vi "CalculateAverageDPARate.vi"(8 "Duration (sec)":dbl, 9 "Period (sec)":dbl, 10 "DPA Rate":dbl, 11 "Total DPA Rate In":dbl) -> (2 "Average DPA Rate":dbl, 3 "Total DPA Rate Out":dbl)   [LabVIEW 2012]
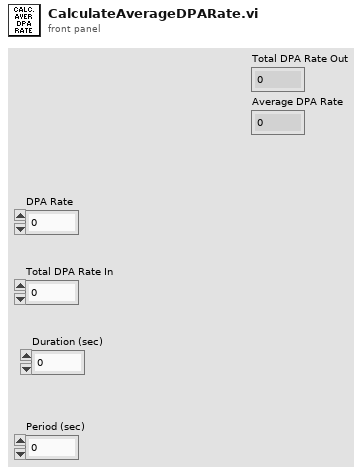
[diagram p1: front panel]
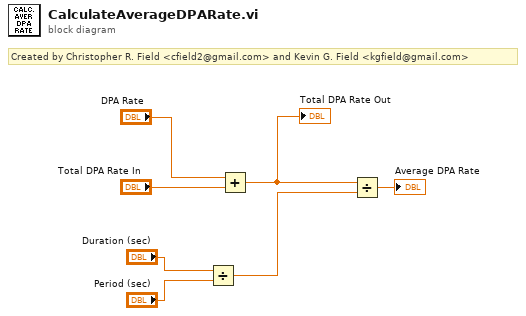
[diagram p0: block diagram]
diagram:
  # "Created by Christopher R. Field <cfield2@gmail.com> and Kevin G. Field <kgfield@gmail.com>"
  n1 = Divide(x="Duration (sec)", y="Period (sec)") -> (x/y=w2:dbl)
  n2 = Add(x="DPA Rate", y="Total DPA Rate In") -> (x+y=w3:dbl)
  "Total DPA Rate Out" <- w3
  n3 = Divide(x=w3, y=w2) -> (x/y=→"Average DPA Rate":dbl)
